vi "read_state.vi"(7 "Enum":T1(ring), 8 "error in":errorcluster, 10 "lines":tag) -> (0 "error out":errorcluster, 2 "data":u8 format="%.0x")   [LabVIEW 2015]
uses:
  <vilib>/DAQmx/read.llb/DAQmx Read (Digital U8 1Chan 1Samp).vi
  <vilib>/DAQmx/create/channels.llb/DAQmx Create Channel (DI-Digital Input).vi
  <vilib>/DAQmx/miscellaneous.llb/DAQmx Fill In Error Info.vi
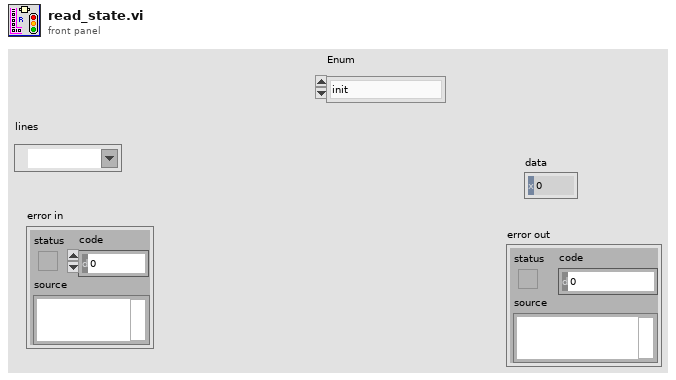
[diagram p1: front panel]
types:
  T1 = enum16{"init", "config", "start", "read", "stop"}
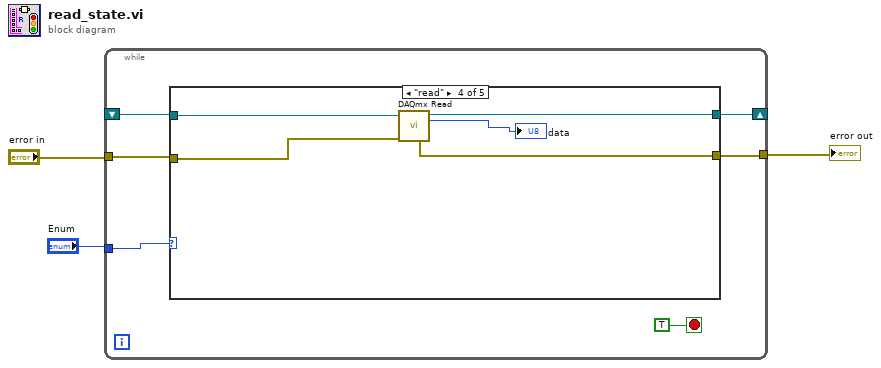
[diagram p0: block diagram]
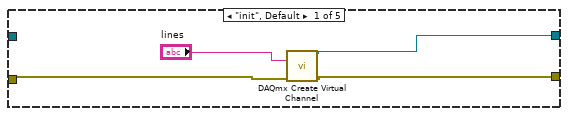
[diagram p2: hidden frame]
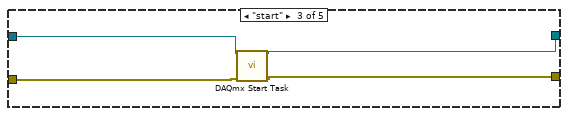
[diagram p4: hidden frame]
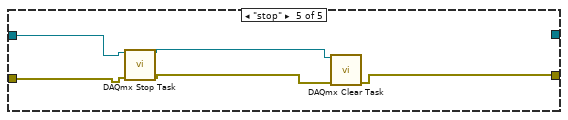
[diagram p5: hidden frame]
diagram:
  n1 = while {
    tunnel: "Enum" -> [w8]
    shift-right: [w7] -> _
    shift-left: _ -> [w6]
    tunnel: "error in" -> [w5]
    tunnel: [w4] -> w1
    stop <- TRUE stop-if-true
    n2 = case shown="\"read\"" w8 {
      tunnel: [w12 w15 w16 w21 _] -> w7
      tunnel: w6 -> [_ w15 w19 w24 w29]
      tunnel: w5 -> [w11 w14 w18 w23 w28]
      tunnel: [w10 w14 w17 w22 w26] -> w4
      frame "init", Default {
        n3 = call-poly <vilib>:"DAQmx Create Virtual Channel.vi"("lines"="lines", "error in"=w11) -> ("task out"=w12:refnum<k21>, "error out"=w10:errorcluster)  [unwired: 12 in]
      }
      frame "config" {
      }
      frame "start" {
        n4 = call <vilib>:"DAQmx Start Task.vi"("task/channels in"=w19, "error in"=w18) -> ("task out"=w16:refnum<k21>, "error out"=w17:errorcluster)  [unwired: 12 in]
      }
      frame "read" {
        n5 = call-poly <vilib>:"DAQmx Read.vi"("task/channels in"=w24, "error in"=w23) -> ("task out"=w21:refnum<k21>, "data"=→"data":u8, "error out"=w22:errorcluster)  [unwired: 11 in]
      }
      frame "stop" {
        n6 = call <vilib>:"DAQmx Stop Task.vi"("task/channels in"=w29, "error in"=w28) -> ("task out"=w27:refnum<k21>, "error out"=w25:errorcluster)  [unwired: 12 in]
        n7 = call <vilib>:"DAQmx Clear Task.vi"("task in"=w27, "error in"=w25) -> ("error out"=w26:errorcluster)  [unwired: 13 in]
      }
    }
  }
  "error out" <- w1
